vi "ListToArray.vi"(1 "delimiter":string, 2 "list":string) -> (0 "Array":string[](array[string]))   [LabVIEW 2009]
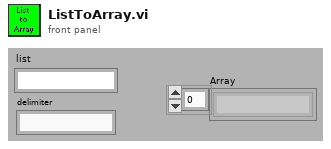
[diagram p1: front panel]
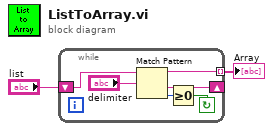
[diagram p0: block diagram]
diagram:
  n1 = while {
    shift-right: [w4] -> _
    shift-left: "list" -> [w8]
    tunnel: [w5] -> w1 mode=indexing
    stop <- w6 continue-if-true
    n2 = Match Pattern(string=w8, regular expression="delimiter") -> (before substring=w5:string, after substring=w4:string, offset past match=w7:i32)  [unwired: 1 in, 1 out]
    n3 = Greater Or Equal To 0?(x=w7) -> (x >= 0?=w6:bool)
  }
  "Array" <- w1
